vi "Protocol.Process J1939 Incoming Messages.vi"(8 "error in":errorcluster, 9 "Active Request?":bool, 10 "CAN frame":T1 {"payload" format="%x"; "timestamp" format="%<%.7X\n%x>T"; "type" items=["CAN Data"=0, "CAN Remote"=1, "CAN Bus Error"=2, "CAN 2.0 Data"=8, "CAN FD Data"=16, "CAN FD+BRS Data"=24, "J1939 Data"=192, "Delay"=224, "Log Trigger"=225, "Start Trigger"=226]; "identifier" format="%x"}, 11 "J1939 Cluster":T3) -> (0 "error out":errorcluster, 3 "J1939 Cluster Out":T3)   [LabVIEW 2015, in "J1939 Addon Engine.lvlib"]
uses:
  J1939 Addon Engine.lvlib
  Types/Protocol.Refs.ctl
  Shared/J1939 Utilities/Types/CAN Outgoing Message Cluster.ctl
  Types/Protocol.RQST Lookup Table Reference.ctl
  Types/Protocol.Address Table Reference.ctl
  <vilib>/xnet/xnet.llb/XNET Frame CAN.ctl
  <vilib>/xnet/xnet.llb/XNET Frame Type CAN.ctl
  Protocol.RQST Lookup Table Act.vi
  Shared/J1939 Utilities/Common Conversions.vi
  Shared/J1939 Utilities/SubVIs/Convert CAN Arb ID to J1939 ID.vi
  Protocol.RQST Look for Response.vi
  Shared/J1939 Utilities/SubVIs/Convert J1939 ID to CAN Arb ID.vi
  Shared/J1939 Utilities/SubVIs/Convert CAN Data (U32) to U8.vi
  Protocol.Get Simulated Previously Active DTCs.vi
  Protocol.Get Simulated Active DTCs.vi
  Shared/J1939 Utilities/Common Messages.vi
  Shared/J1939 Utilities/SubVIs/Acknowledgement.vi
  Protocol.Send Reset Previously Active DTC to Main.vi
  Protocol.Send Reset Active DTC to Main.vi
  Protocol.Convert Signals to Frame by ID.vi
  Protocol.Address Lookup Table Action.vi
  Protocol.Parse Message Type.vi
  Protocol.Convert Data to DTC Frame.vi
  Protocol.Address Lookup Table.vi
  <vilib>/xnet/xnet.llb/XNET Clear.vi
  <vilib>/xnet/xnet.llb/XNET Convert.vi
  <vilib>/xnet/xnet.llb/XNET Convert (Signal to Frame CAN).vi
  <vilib>/xnet/xnet.llb/XNET Create Session.vi
  <vilib>/xnet/xnet.llb/XNET Create Session (Conversion).vi
  Protocol.RQST Lookup Table.vi
  Shared/J1939 Utilities/J1939 Utilities.lvlib
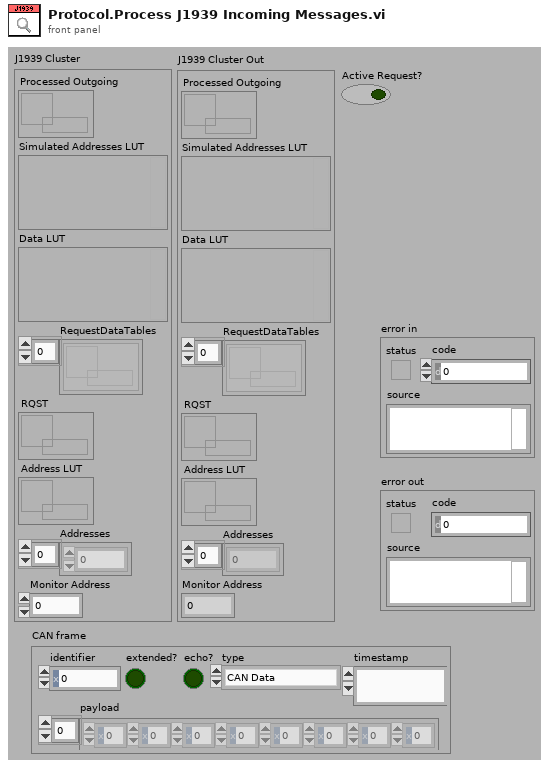
[diagram p1: front panel]
types:
  T1 = typedef "XNET Frame CAN.ctl" = cluster{"timestamp":timestamp, "payload":u8[], "identifier":u32, "type":T2, "extended?":bool, "echo?":bool}
  T2 = typedef "XNET Frame Type CAN.ctl" = u8
  T3 = typedef "J1939 Addon Engine.lvlib/Protocol.Refs.ctl" = cluster{"Processed Outgoing":refnum<queue>, "Simulated Addresses LUT":variant, "Data LUT":variant, "RequestDataTables":refnum<k33>[], "RQST":T4, "Address LUT":T5, "Addresses":u8[], "Monitor Address":u8}
  T4 = typedef "J1939 Addon Engine.lvlib/Protocol.RQST Lookup Table Reference.ctl" = refnum<data-value>
  T5 = typedef "J1939 Addon Engine.lvlib/Protocol.Address Table Reference.ctl" = refnum<data-value>
  T6 = typedef "J1939 Addon Shared.lvlib/J1939 Utilities.lvlib/Message Types.ctl" = enum8{"PDU 1", "RQST2", "XFER", "ACKM", "RQST", "TP.DT - RTS/CTS", "TP.DT - BAM", "TP.CM - RTS", "TP.CM - CTS", "TP.CM - EndofMsgACK", "TP.CM - BAM", "TP.CM - Abort", "TP.CM - Error", "ACL", "Proprietary A", "PDU 2", "Proprietary B", "Error"}
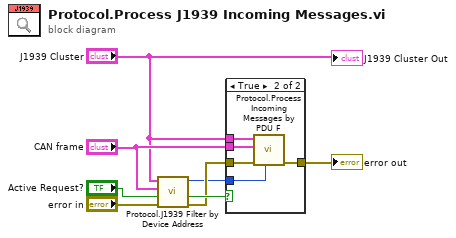
[diagram p0: block diagram]
diagram:
  n1 = call "Protocol.J1939 Filter by Device Address.vi"("error in"="error in", "Active Request?"="Active Request?", "CAN Frame"="CAN frame", "J1939 Cluster"="J1939 Cluster") -> ("error out"=w2:errorcluster, "Pass Through"=w3:bool, "State"=w1:T6)  [unwired: 5 in]
  n2 = case shown="True" w3 {
    tunnel: [w9 w14] -> w8
    tunnel: w2 -> [w9 w13]
    tunnel: "CAN frame" -> [_ w12]
    tunnel: "J1939 Cluster" -> [_ w10]
    tunnel: w1 -> [_ w11]
    frame False {
    }
    frame True {
      n3 = call "Protocol.Process Incoming Messages by PDU F.vi"("State"=w11, "error in"=w13, "CAN frame"=w12, "J1939 Cluster"=w10) -> ("error out"=w14:errorcluster)  [unwired: 7 in]
    }
  }
  "error out" <- w8
  "J1939 Cluster Out" <- "J1939 Cluster"
